vi "Test T-Cube.vi"() -> ()   [LabVIEW 2026]
uses:
  C:/Users/flepetit/Desktop/Projet BTS Photonique/Thorlabs.MotionControl.TCube.PiezoCLI.dll
  Thorlabs.MotionControl.TCube.PiezoCLI.dll
  C:/Users/flepetit/Desktop/Projet BTS Photonique/Thorlabs.MotionControl.Controls.dll
  Thorlabs.MotionControl.Controls.dll
panel:
  out "GetOutputVoltage":dbl
  in  "stop":bool
  out "CloseDevice":bool
  out "CreateDevice":bool
  in  "TCubePiezoControl":refnum<k24>(container)
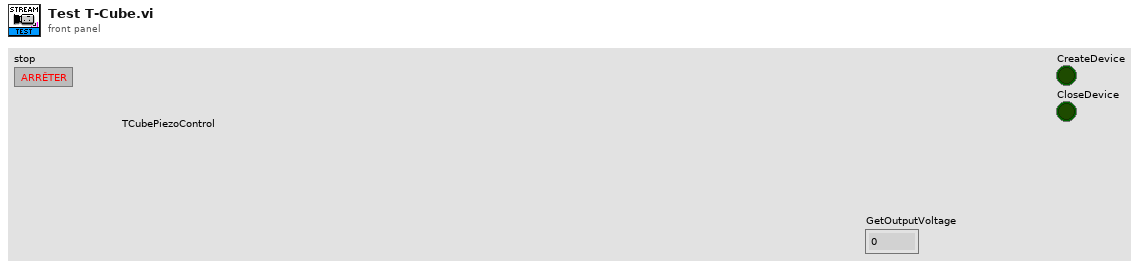
[diagram p1: front panel]
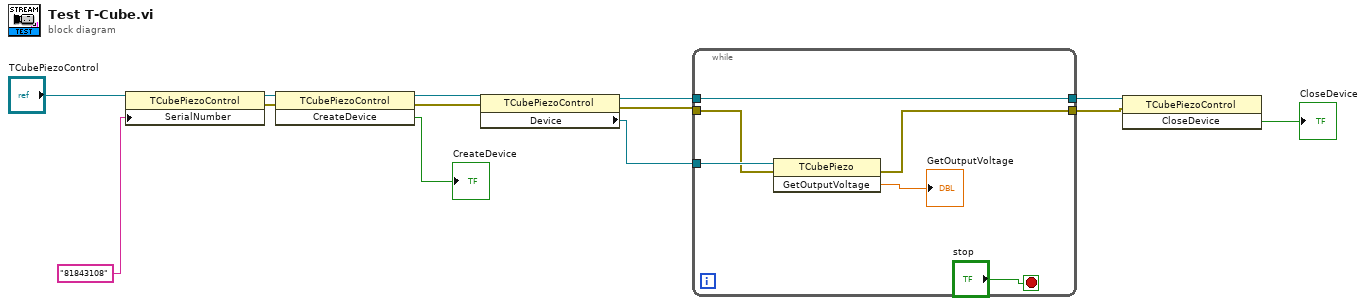
[diagram p0: block diagram]
diagram:
  n1 = property class="TCubePiezoControl"(reference="TCubePiezoControl", "SerialNumber"="81843108") -> (reference out=w12:refnum<k24>, error out=w11:errorcluster)  [unwired: 1 in]
  n2 = invoke class="TCubePiezoControl" method="CreateDevice"(reference=w12, error in=w11) -> (reference out=w5:refnum<k24>, error out=w4:errorcluster, "CreateDevice"=→"CreateDevice":bool)  [unwired: 1 in]
  n3 = property class="TCubePiezoControl"(reference=w5, error in=w4) -> (reference out=w2:refnum<k24>, error out=w3:errorcluster, "Device"=w1:refnum<k24>)
  n4 = while {
    tunnel: [w18] -> w7
    tunnel: w2 -> [w18]
    tunnel: [w15] -> w6
    tunnel: w3 -> [w16]
    tunnel: w1 -> [w17]
    stop <- "stop" stop-if-true
    n5 = invoke class="TCubePiezo" method="GetOutputVoltage"(reference=w17, error in=w16) -> (error out=w15:errorcluster, "GetOutputVoltage"=→"GetOutputVoltage":dbl)  [unwired: 1 in, 1 out]
  }
  n6 = invoke class="TCubePiezoControl" method="CloseDevice"(reference=w7, error in=w6) -> ("CloseDevice"=→"CloseDevice":bool)  [unwired: 1 in, 2 out]
